vi "Signal Analysis using filters.vi"() -> ()   [LabVIEW 2024]
panel:
  out "Filtered signal":dynamicdata(graph)
  in  "Low pass value":dbl
  in  "stop":bool
  out "Simulate signal":dynamicdata(graph)
  # "Overview: Signal analysis using low pass filter and  using the filter  we can remove the noise from the signals by providing the frequency.\n\nInstructions:\n1. Give the Low pass value.\n2. Run the VI."
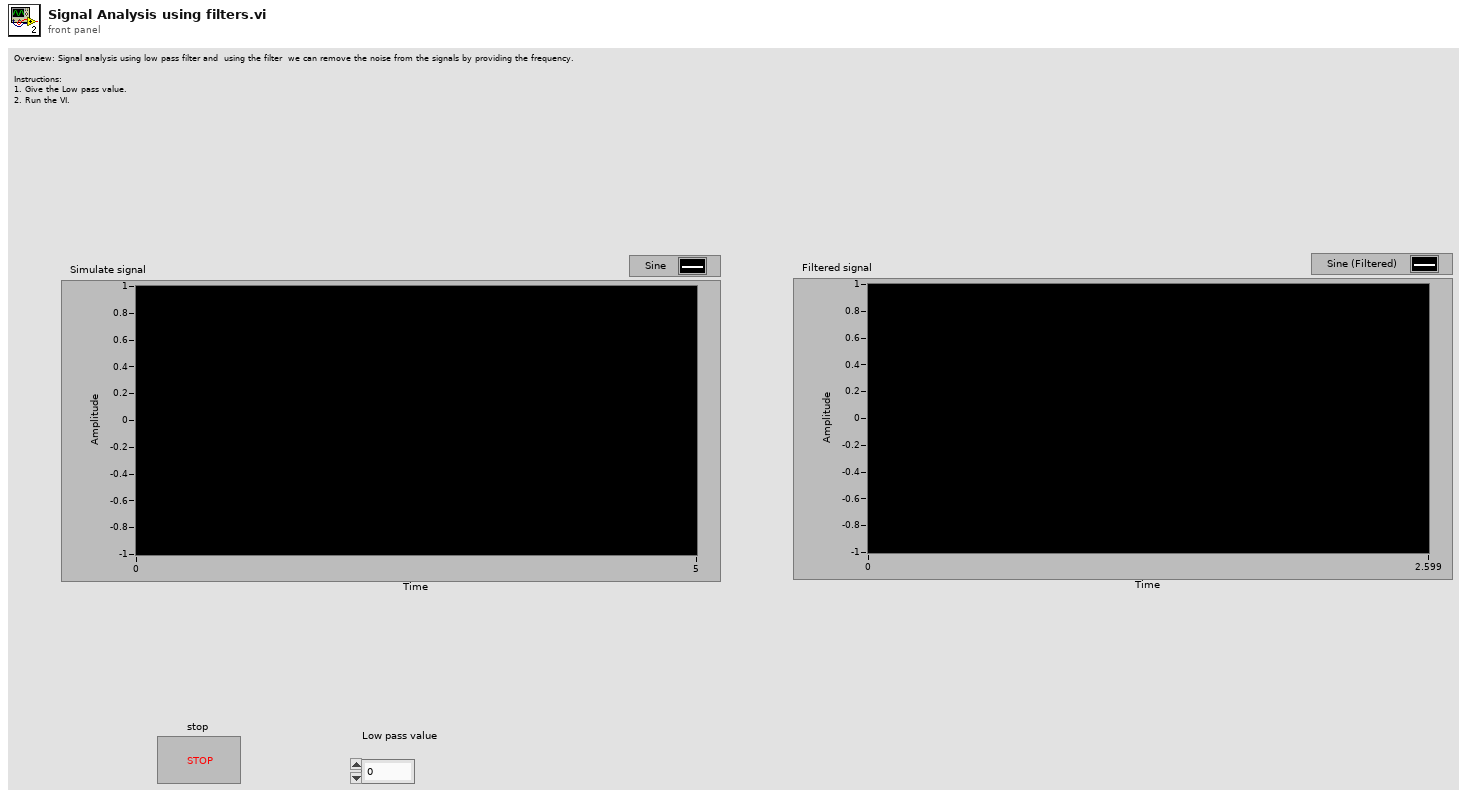
[diagram p1: front panel]
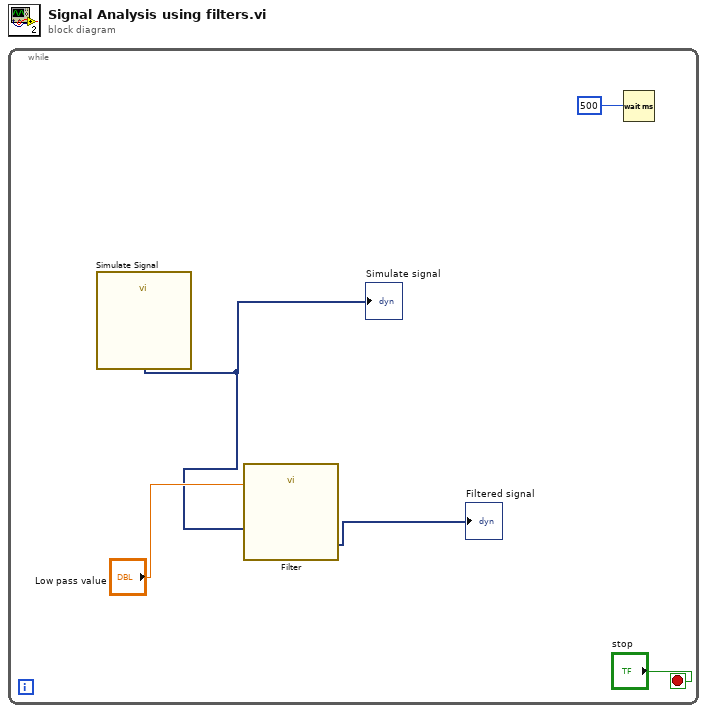
[diagram p0: block diagram]
diagram:
  n1 = while {
    stop <- "stop" stop-if-true
    n2 = call "Simulate Signal"() -> ("Sine"=w2:dynamicdata)  [unwired: 14 in, 1 out]
    "Simulate signal" <- w2
    n3 = call "Filter"("Lower Cut-Off"="Low pass value", "Signal"=w2) -> ("Filtered Signal"=→"Filtered signal":dynamicdata)  [unwired: 8 in, 1 out]
    n4 = Wait (ms)(milliseconds to wait=u32 500) -> ()  [unwired: 1 out]
  }
